vi "WriteIO.fpga.vi"(10 "x (in)":u32, 11 "Memory (in)":refnum<k21>="OutputMatrix2") -> (2 "x (out)":u32)   [LabVIEW 2012]
uses:
  <vilib>/rvi/DataTransferAndStorage/Container/Common/niFpgaContainerExecOnDevCompGetState.vi
  <vilib>/rvi/DataTransferAndStorage/Container/Common/niFpgaContainerGetUniqueNameForEmu.vi
  <vilib>/rvi/Memory/Memory_Emulation/niFpgaMemoryEmulationCacheClearOnFirstRun.vi
  <vilib>/rvi/Memory/Memory_Emulation/nirvimemoryEmulationManagerCache_MakeExclusive.vi
  <vilib>/rvi/Memory/Memory_Emulation/niFpgaMemoryEmulationValidateCache.vi
  <vilib>/rvi/Memory/Memory_Emulation/nirvimemoryEmulationManagerCache_ReleaseExclusive.vi
  <vilib>/rvi/Memory/Memory_Emulation/nirvimemoryEmulationManagerCache_InsertValue.vi
  <vilib>/Utility/error.llb/Clear Errors.vi
  <vilib>/rvi/Memory/Memory_Emulation/nirvimemoryEmulationManagerCache_GetValue.vi
  <vilib>/rvi/eio/common/nirviEmuTemplateMethod_errors.vi
  <vilib>/rvi/DataTransferAndStorage/Container/XNode/niFpgaContainer.xnode
  <vilib>/rvi/Memory/Memory_Emulation/niFpgaMemoryEmulationRefIn.vi
  <vilib>/eio/EIONode/EIONode.xnode
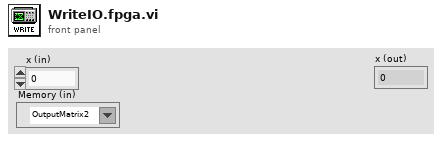
[diagram p1: front panel]
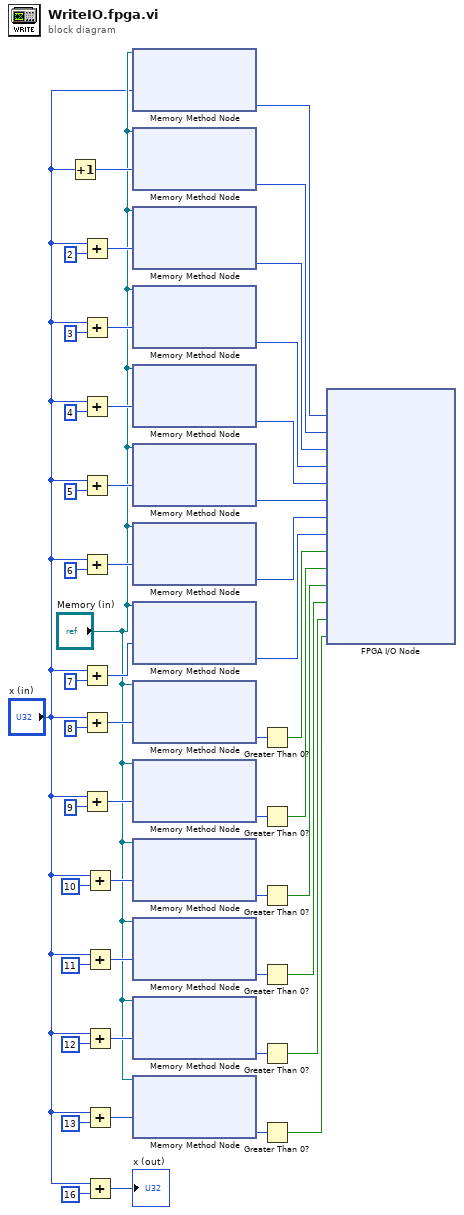
[diagram p0: block diagram]
diagram:
  n1 = Increment(x="x (in)") -> (x+1=w29:u32)
  n2 = Add(x="x (in)", y=u32 2) -> (x+y=w25:u32)
  n3 = Add(x="x (in)", y=u32 3) -> (x+y=w26:u32)
  n4 = Add(x="x (in)", y=u32 4) -> (x+y=w22:u32)
  n5 = Add(x="x (in)", y=u32 5) -> (x+y=w20:u32)
  n6 = Add(x="x (in)", y=u32 6) -> (x+y=w18:u32)
  n7 = Add(x="x (in)", y=u32 7) -> (x+y=w16:u32)
  n8 = Add(x="x (in)", y=u32 8) -> (x+y=w13:u32)
  n9 = Add(x="x (in)", y=u32 9) -> (x+y=w15:u32)
  n10 = Add(x="x (in)", y=u32 10) -> (x+y=w11:u32)
  n11 = Add(x="x (in)", y=u32 11) -> (x+y=w9:u32)
  n12 = Add(x="x (in)", y=u32 12) -> (x+y=w5:u32)
  n13 = Add(x="x (in)", y=u32 13) -> (x+y=w6:u32)
  n14 = Add(x="x (in)", y=u32 16) -> (x+y=→"x (out)":u32)
  n15 = xnode ("Memory Method Node")("Address"="x (in)", "Memory In"="Memory (in)") -> ("Data"=w49:i16)  [unwired: 1 out]
  n16 = xnode ("Memory Method Node")("Address"=w29, "Memory In"="Memory (in)") -> ("Data"=w48:i16)  [unwired: 1 out]
  n17 = xnode ("Memory Method Node")("Address"=w25, "Memory In"="Memory (in)") -> ("Data"=w47:i16)  [unwired: 1 out]
  n18 = xnode ("Memory Method Node")("Address"=w26, "Memory In"="Memory (in)") -> ("Data"=w46:i16)  [unwired: 1 out]
  n19 = xnode ("Memory Method Node")("Address"=w22, "Memory In"="Memory (in)") -> ("Data"=w45:i16)  [unwired: 1 out]
  n20 = xnode ("Memory Method Node")("Address"=w20, "Memory In"="Memory (in)") -> ("Data"=w44:i16)  [unwired: 1 out]
  n21 = xnode ("Memory Method Node")("Address"=w18, "Memory In"="Memory (in)") -> ("Data"=w43:i16)  [unwired: 1 out]
  n22 = xnode ("Memory Method Node")("Address"=w16, "Memory In"="Memory (in)") -> ("Data"=w42:i16)  [unwired: 1 out]
  n23 = xnode ("Memory Method Node")("Address"=w13, "Memory In"="Memory (in)") -> ("Data"=w41:i16)  [unwired: 1 out]
  n24 = xnode ("Memory Method Node")("Address"=w15, "Memory In"="Memory (in)") -> ("Data"=w39:i16)  [unwired: 1 out]
  n25 = xnode ("Memory Method Node")("Address"=w11, "Memory In"="Memory (in)") -> ("Data"=w38:i16)  [unwired: 1 out]
  n26 = xnode ("Memory Method Node")("Address"=w9, "Memory In"="Memory (in)") -> ("Data"=w37:i16)  [unwired: 1 out]
  n27 = xnode ("Memory Method Node")("Address"=w5, "Memory In"="Memory (in)") -> ("Data"=w36:i16)  [unwired: 1 out]
  n28 = xnode ("Memory Method Node")("Address"=w6, "Memory In"="Memory (in)") -> ("Data"=w31:i16)  [unwired: 1 out]
  n29 = Greater Than 0?(x=w41) -> (x > 0?=w40:bool)
  n30 = Greater Than 0?(x=w39) -> (x > 0?=w35:bool)
  n31 = Greater Than 0?(x=w38) -> (x > 0?=w34:bool)
  n32 = Greater Than 0?(x=w37) -> (x > 0?=w33:bool)
  n33 = Greater Than 0?(x=w36) -> (x > 0?=w32:bool)
  n34 = Greater Than 0?(x=w31) -> (x > 0?=w30:bool)
  n35 = xnode "FPGA I/O Node"("Connector0/AO0"=w49, "Connector0/AO1"=w48, "Connector0/AO2"=w47, "Connector0/AO3"=w46, "Connector0/AO4"=w45, "Connector0/AO5"=w44, "Connector0/AO6"=w43, "Connector0/AO7"=w42, "Connector0/DIO0"=w40, "Connector0/DIO1"=w35, "Connector0/DIO2"=w34, "Connector0/DIO3"=w33, "Connector0/DIO4"=w32, "Connector0/DIO5"=w30) -> ()  [unwired: 14 in, 14 out]
